vi "Load Images from File.vi"(4 "frame":i32, 6 "Force Load":bool, 8 "Images":i32, 9 "image files":string[](array[string]), 10 "Folder Location":path, 11 "Refnum in":T1) -> (0 "error out":errorcluster, 2 "Number of Frames":i32, 3 "Refnum out":T1)   [LabVIEW 2019]
uses:
  <vilib>/vision/Image Controls.llb/IMAQ Image.ctl
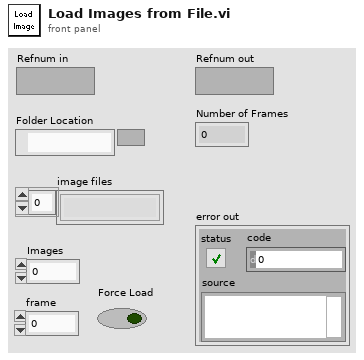
[diagram p1: front panel]
types:
  T1 = typedef "IMAQ Image.ctl" = refnum<image>
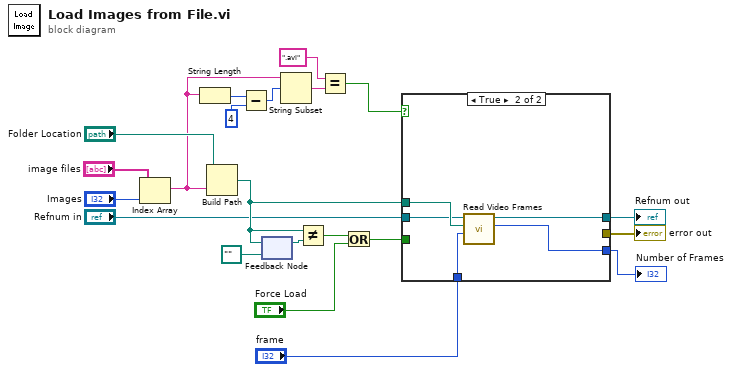
[diagram p0: block diagram]
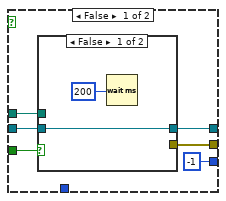
[diagram p2: hidden frame]
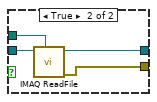
[diagram p3: hidden frame]
diagram:
  n1 = Index Array(array="image files", index="Images") -> (element=w9:string)
  n2 = String Length(string=w9) -> (length=w8:i32)
  n3 = Build Path(base path="Folder Location", name or relative path=w9) -> (appended path=w20:path)
  n4 = Subtract(x=w8, y=4) -> (x-y=w7:i32)
  n5 = feedback #1(path "" ("appended path")) -> (w18:path)
  n6 = feedback-in #1(w20) -> ()
  n7 = String Subset(string=w9, offset (0)=w7) -> (substring=w4:string)  [unwired: 1 in]
  n8 = Not Equal?(x=w20, y=w18) -> (x != y?=w11:bool)
  n9 = Equal?(x=".avi", y=w4) -> (x = y?=w3:bool)
  n10 = Or(x=w11, y="Force Load") -> (x .or. y?=w10:bool)
  n11 = case shown="True" w3 {
    tunnel: w20 -> [w27 w38]
    tunnel: "Refnum in" -> [w26 w37]
    tunnel: [w25 _] -> w14
    tunnel: [w24 w36] -> w13
    tunnel: w10 -> [w23 _]
    tunnel: [-1 ("Number of Frames") w35] -> w2
    tunnel: "frame" -> [_ w34]
    frame False {
      n12 = case shown="False" w23 {
        tunnel: [w29 w33] -> w24
        tunnel: [_ w32] -> w25
        tunnel: w26 -> [w29 w31]
        tunnel: w27 -> [_ w30]
        frame False {
          n13 = Wait (ms)(milliseconds to wait=u32 200 ("delay (ms)")) -> ()  [unwired: 1 out]
        }
        frame True {
          n14 = call "IMAQ ReadFile"("File Path"=w30, "Image"=w31) -> ("error out"=w32:errorcluster, "Image Out"=w33:T1)  [unwired: 5 in, 3 out]
        }
      }
    }
    frame True {
      n15 = call "Read Video Frames.vi"("frame"=w34, "Path"=w38, "Refnum in"=w37) -> ("Number of Frames"=w35:i32, "Refnum out"=w36:T1)  [unwired: 7 in]
    }
  }
  "error out" <- w14
  "Refnum out" <- w13
  "Number of Frames" <- w2
